vi "RunningAverage-AddSection.vi"(8 "Error in":errorcluster, 11 "Custom Device ref":T1 format="%.0x") -> (0 "Error out":errorcluster, 3 "Custom Device ref out":T1 format="%.0x")   [LabVIEW 2014, in "Waveform-Processing-Custom-Device Shared.lvlib" / "Running Average.lvlib"]
uses:
  Running Average.lvlib
  <vilib>/NI Veristand/Custom Device API/Custom Device Item Ref.ctl
  <vilib>/NI Veristand/Custom Device API/Custom Device Channel.ctl
  <vilib>/NI Veristand/Custom Device API/Custom Device Channel Type.ctl
  Constants.vi
  <vilib>/NI Veristand/Custom Device API/Set Item Property (Dependent Node Pointer).vi
  <vilib>/NI Veristand/Custom Device API/Custom Device API.lvlib
  Waveform-Processing-Custom-Device Shared.lvlib
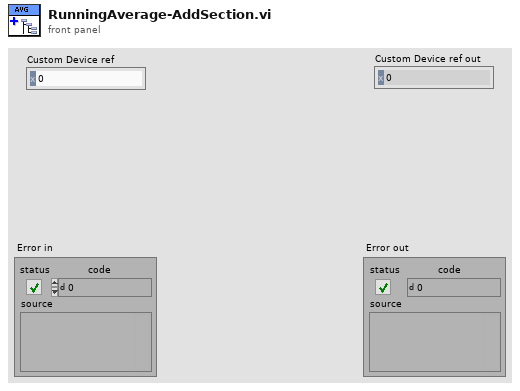
[diagram p1: front panel]
types:
  T1 = typedef "Custom Device API.lvlib/Custom Device Item Ref.ctl" = u64
  T2 = typedef "Custom Device API.lvlib/Custom Device Channel.ctl" = cluster{"Type":T3, "Units":string, "Default Value":dbl, "Faultable":bool, "Scalable":bool}
  T3 = typedef "Custom Device API.lvlib/Custom Device Channel Type.ctl" = enum16{"Input", "Output"}
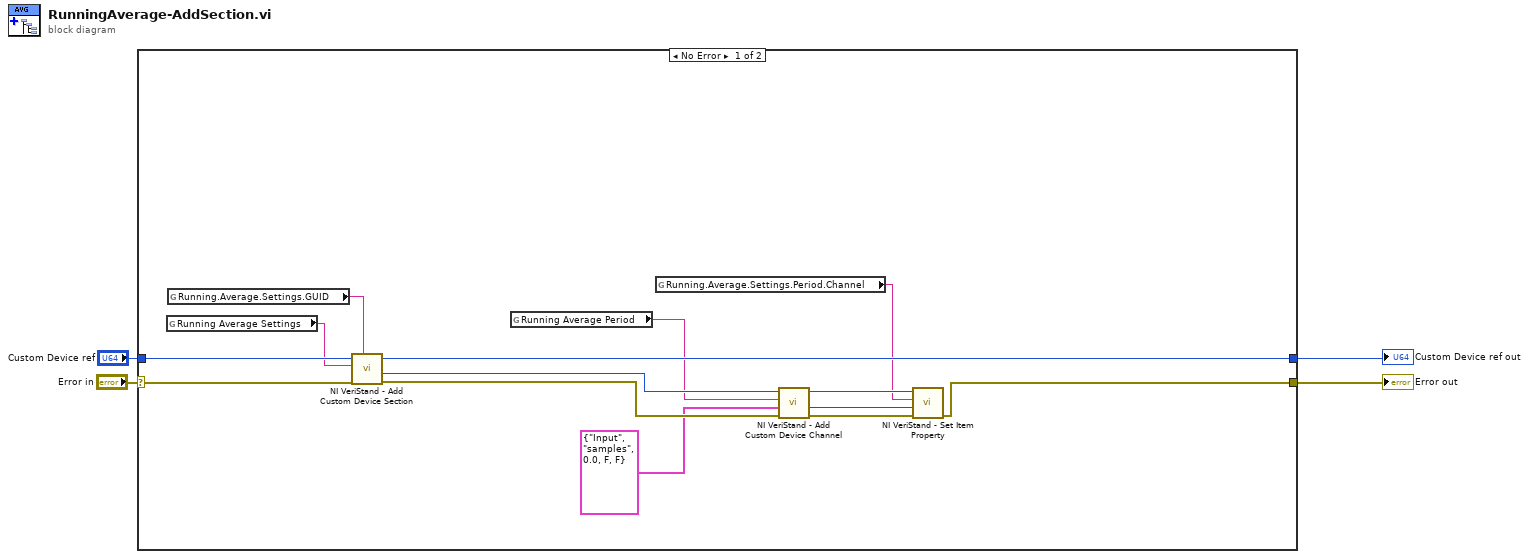
[diagram p0: block diagram]
diagram:
  n1 = case shown="No Error" "Error in" {
    selector: "Error in" -> [w18 w20]
    tunnel: "Custom Device ref" -> [w17 w19]
    tunnel: [w5 w20] -> w2
    tunnel: [w12 w19] -> w1
    frame No Error {
      n2 = global read "Constants.vi" "Running Average Settings"() -> (w16:string)
      n3 = global read "Constants.vi" "Running.Average.Settings.GUID"() -> (w15:string)
      n4 = call <vilib>:"NI VeriStand - Add Custom Device Section.vi"("GUID (Default Section)"=w15, "error in (no error)"=w18, "Section Name"=w16, "Parent Ref in"=w17) -> ("error out"=w14:errorcluster, "Section Ptr"=w13:T1, "Parent Ref out"=w12:T1)  [unwired: 4 in, 1 out]
      n5 = global read "Constants.vi" "Running Average Period"() -> (w11:string)
      n6 = global read "Constants.vi" "Running.Average.Settings.Period.Channel"() -> (w6:string)
      n7 = call <vilib>:"NI VeriStand - Add Custom Device Channel.vi"("error in (no error)"=w14, "Channel"=T2 {"Type"=enum."Input", "Units"="samples", "Default Value"=0.0, "Faultable"=FALSE, "Scalable"=FALSE}, "Channel Name"=w11, "Parent Ref in"=w13) -> ("error out"=w7:errorcluster, "Channel Ref"=w8:T1, "Parent Ref out"=w9:T1)  [unwired: 4 in, 1 out]
      n8 = call-poly <vilib>:"NI VeriStand - Set Item Property.vi"("error in (no error)"=w7, "Dependent Node Ref"=w8, "Property Name"=w6, "Item Ref in"=w9) -> ("error out"=w5:errorcluster)  [unwired: 5 in, 2 out]
    }
    frame Error {
    }
  }
  "Error out" <- w2
  "Custom Device ref out" <- w1
